vi "BRig_dataLC_init.vi"() -> (3 "output_dataLC":u16[](array[numeric]))   [LabVIEW 2014]
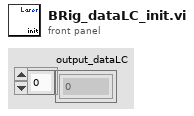
[diagram p1: front panel]
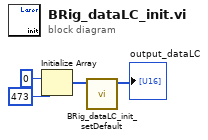
[diagram p0: block diagram]
diagram:
  n1 = Initialize Array(u16 0 ("element"), 473 ("dimension size")) -> (w2:u16[])
  n2 = call "BRig_dataLC_init_setDefault.vi"("input_dataLC"=w2) -> ("output_dataLC"=→"output_dataLC":u16[])  [unwired: 10 in]
